vi "H5Tlock.vi"(6 "error in (no error)":errorcluster, 9 "HDF5Type  Ref":T1) -> (0 "error out":errorcluster, 3 "HDF5 Type Ref out":T1)   [LabVIEW 2017]
doc: "Locks a datatype."
uses:
  <vilib>/UPVI/lvhdf5/library.llb/HDF5 Ref.ctl
  <vilib>/UPVI/lvhdf5/hdf5.dll
panel:
  # "LVHDF5 Toolkit\nCopyright (c) 2005-2013 by Jason D. Sommerville\nCopyright (c) 2014 by UPVI, LLC.\n\nThis use and distribution of this file is governed by the terms found in \nLICENSE.txt distributed with this toolkit and installed at\n <user.lib>\\_lvhdf5\\LICENSE.txt"
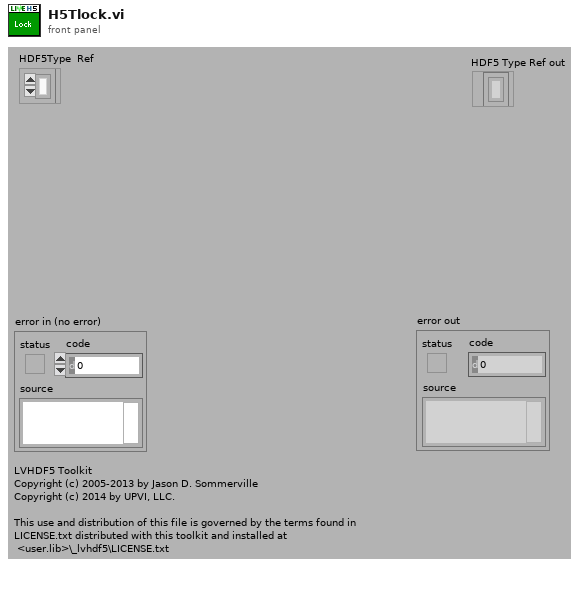
[diagram p1: front panel]
types:
  T1 = typedef "HDF5 Ref.ctl" = refnum<k1>
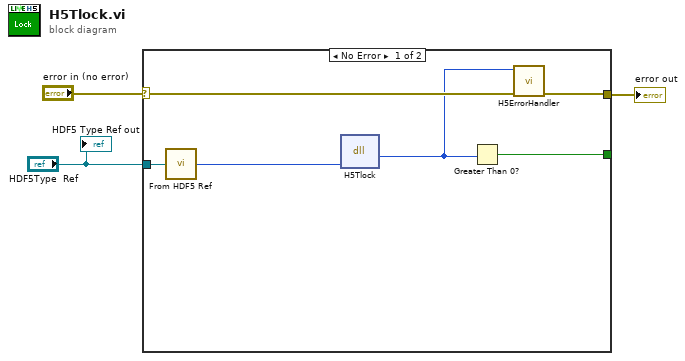
[diagram p0: block diagram]
diagram:
  n1 = case shown="No Error" "error in (no error)" {
    selector: "error in (no error)" -> [w9 w10]
    tunnel: [w8 w10] -> w2
    tunnel: "HDF5Type  Ref" -> [w7 _]
    tunnel: [w4 _] -> _
    frame No Error {
      n2 = call <vilib>:"From HDF5 Ref.vi"("HDF5 Ref"=w7) -> ("I32"=w6:i32)
      n3 = dll-call lib="C:/Program Files/National Instruments/LabVIEW 2017/vi.lib/UPVI/lvhdf5/hdf5.dll" fn="H5Tlock"("loc_id"=w6) -> (w5:i32)  [unwired: 4 in, 2 out]
      n4 = Greater Than 0?(x=w5) -> (x > 0?=w4:bool)
      n5 = call <vilib>:"H5ErrorHandler.vi"("error in (no error)"=w9, "herr_t"=w5) -> ("error out"=w8:errorcluster)  [unwired: 3 in, 4 out]
    }
    frame Error {
    }
  }
  "error out" <- w2
  "HDF5 Type Ref out" <- "HDF5Type  Ref"
